vi "Mexa parse.vi"(10 "Byte array":u8[](array[numeric])=[6, 64, 24, 31, 2, 255, 167, 0, 3, 255, 54, 0, 0, 3, 231, 39, 15, 3, 234, 0, 21, 0, 0, 0, 0, 0, 0, 129]) -> (2 "Output":dbl[](array[numeric]))   [LabVIEW 2014]
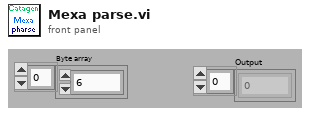
[diagram p1: front panel]
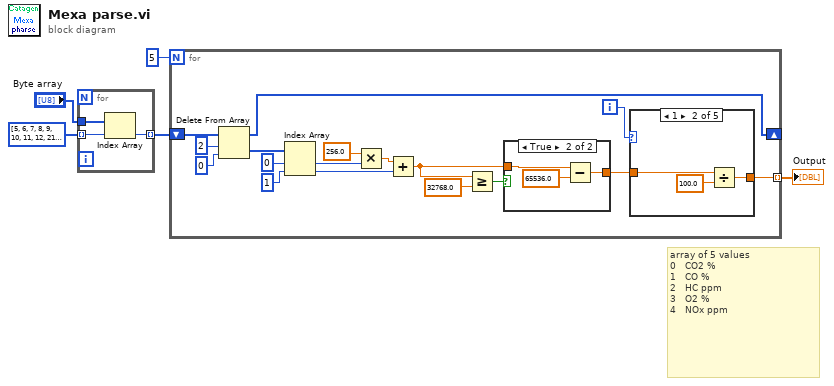
[diagram p0: block diagram]
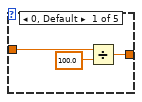
[diagram p2: hidden frame]
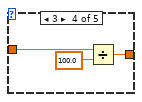
[diagram p4: hidden frame]
diagram:
  # "array of 5 values\n0   CO2 %\n1   CO %\n2   HC ppm\n3   O2 %\n4   NOx ppm"
  n1 = for {
    tunnel: "Byte array" -> [w8]
    tunnel: i32[] [5, 6, 7, 8, 9, 10, 11, 12, 21, 22] -> [w7] mode=indexing
    tunnel: [w6] -> w3 mode=indexing
    n2 = Index Array(array=w8, index=w7) -> (element=w6:u8)
  }
  n3 = for {
    N: 5 -> [_]
    shift-right: [w19] -> _
    shift-left: w3 -> [w25]
    tunnel: [w9] -> w1 mode=indexing
    i -> [w11]
    n4 = Delete From Array(array=w25, length=2, index=0) -> (deleted portion=w22:u8[], array with subset deleted=w19:u8[])
    n5 = Index Array(array=w22, index #1=0 ("index"), index #2=1 ("index")) -> (element #1=w17:u8, element #2=w15:u8)
    n6 = Multiply(x=256.0, y=w17) -> (x*y=w16:dbl)
    n7 = Add(x=w16, y=w15) -> (x+y=w12:dbl)
    n8 = Greater Or Equal?(x=w12, y=32768.0) -> (x >= y?=w14:bool)
    n9 = case shown="True" w14 {
      tunnel: w12 -> [w37 w40]
      tunnel: [w37 w39] -> w10
      frame False {
      }
      frame True {
        n10 = Subtract(x=w40, y=65536.0) -> (x-y=w39:dbl)
      }
    }
    n11 = case shown="1" w11 {
      tunnel: w10 -> [w28 w29 w32 w33 w36]
      tunnel: [w26 w30 w32 w34 w36] -> w9
      frame 0, Default {
        n12 = Divide(x=w28, y=100.0) -> (x/y=w26:dbl)
      }
      frame 1 {
        n13 = Divide(x=w29, y=100.0) -> (x/y=w30:dbl)
      }
      frame 2 {
      }
      frame 3 {
        n14 = Divide(x=w33, y=100.0) -> (x/y=w34:dbl)
      }
      frame 4 {
      }
    }
  }
  "Output" <- w1
